vi "CreateRequestTable.vi"() -> ()   [LabVIEW 2015]
uses:
  TypeDef/RequestsTableDbTableName.ctl
  TypeDef/RequestsTableColumnNames.ctl
  <vilib>/addons/database/Auxilliary.llb/DB Tools DataTypes.ctl
  <vilib>/addons/database/Auxilliary.llb/DB Tools Column Info.ctl
  <vilib>/addons/database/Connection.llb/DB Tools Open Connec (Path).vi
  <vilib>/addons/database/NI_Database_API.lvlib
panel:
  in  "table":T1="RequestTable"
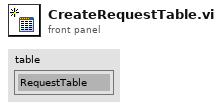
[diagram p1: front panel]
types:
  T1 = typedef "RequestsTableDbTableName.ctl" = string
  T2 = typedef "NI_Database_API.lvlib/DB Tools DataTypes.ctl" = enum16{"String", "Long (I32)", "Single (SGL)", "Double (DBL)", "Date/Time", "Binary"}
  T3 = typedef "RequestsTableColumnNames.ctl" = string[]
  T4 = typedef "NI_Database_API.lvlib/DB Tools Column Info.ctl" = cluster{"column name":string, "data type":T2, "size":i32, "allow null?":bool}
  T5 = typedef "NI_Database_API.lvlib/Conn ObjectReference.ctl" = refnum<k1>
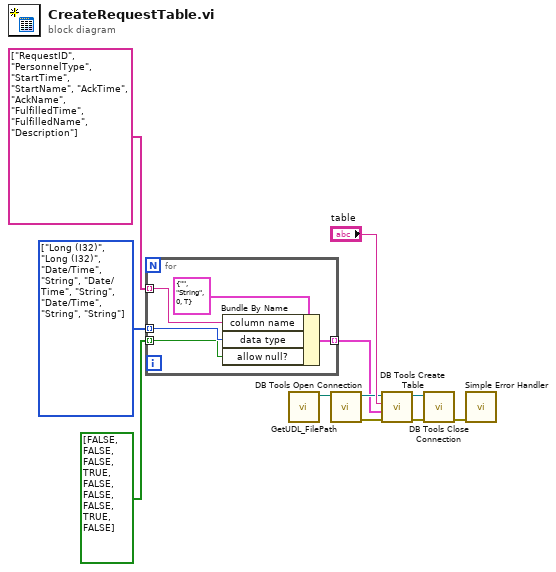
[diagram p0: block diagram]
diagram:
  w4 = T2[] [enum."Long (I32)", enum."Long (I32)", enum."Date/Time", enum."String", enum."Date/Time", enum."String", enum."Date/Time", enum."String", enum."String"] items=["String", "Long (I32)", "Single (SGL)", "Double (DBL)", "Date/Time", "Binary"] ("Array")
  n1 = for {
    tunnel: T3 ["RequestID", "PersonnelType", "StartTime", "StartName", "AckTime", "AckName", "FulfilledTime", "FulfilledName", "Description"] ("Array") -> [w15] mode=indexing
    tunnel: w4 -> [w14] mode=indexing
    tunnel: bool[] [FALSE, FALSE, FALSE, TRUE, FALSE, FALSE, FALSE, TRUE, FALSE] ("Array") -> [w13] mode=indexing
    tunnel: [w12] -> w2 mode=indexing
    n2 = Bundle By Name(cluster=T4 {"column name"="", "data type"=enum."String", "size"=0, "allow null?"=TRUE} ("column information"), "column name"=w15, "data type"=w14, "allow null?"=w13) -> (w12:T4)
  }
  n3 = call "GetUDL_FilePath.vi"() -> ("UDL file path"=w1:path)  [unwired: 11 in]
  n4 = call-poly <vilib>:"DB Tools Open Connection.vi"("connection information"=w1) -> ("error out"=w9:errorcluster, "connection reference"=w8:T5)  [unwired: 7 in]
  n5 = call <vilib>:"DB Tools Create Table.vi"("error in (no error)"=w9, "column information"=w2, "table"="table", "connection reference"=w8) -> ("error out"=w7:errorcluster, "connection reference out"=w6:T5)  [unwired: 4 in]
  n6 = call <vilib>:"DB Tools Close Connection.vi"("error in (no error)"=w7, "connection reference"=w6) -> ("error out"=w10:errorcluster)  [unwired: 5 in]
  n7 = call <vilib>:"Simple Error Handler.vi"("error in (no error)"=w10) -> ()  [unwired: 4 in, 5 out]
